vi "ARCO Read Client.vi"() -> ()   [LabVIEW 2017]
uses:
  <vilib>/OPCUA/controls/NodeIds.ctl
  <vilib>/OPCUA/controls/NodeId.ctl
  <vilib>/OPCUA/NI OPC UA Client.lvlib
panel:
  in  "stop":bool
  out "error out":errorcluster
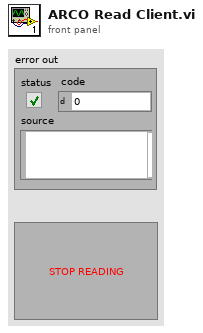
[diagram p1: front panel]
types:
  T1 = cluster{"message mode":enum16{"None", "Sign", "Sign and Encrypt"}, "security":enum16{"Basic256", "Basic128Rsa15"}}
  T2 = typedef "NodeIds.ctl" = T3[]
  T3 = typedef "NodeId.ctl" = string
  T4 = typedef "OPC UA Client Refnum.ctl" = refnum<k21>
  T5 = typedef "Subscription ID.ctl" = u32
  T6 = typedef "Subscription Data Change.ctl" = cluster{"node ID":T3, " value":variant, "timestamp":timestamp, "data type":T7, "status code":T8}
  T7 = typedef "Data Type.ctl" = u16
  T8 = typedef "OPC UA StatusCode.ctl" = u32
  T9 = cluster{"[0]":sgl, "[1]":sgl, "[2]":sgl, "[3]":sgl, "[4]":sgl, "[5]":sgl, "[6]":sgl, "[7]":sgl, "[8]":sgl, "[9]":sgl, "[10]":sgl, "[11]":sgl, "[12]":sgl, "[13]":sgl, "[14]":sgl, "[15]":sgl, "[16]":sgl, "[17]":sgl, "[18]":sgl, "[19]":sgl, "[20]":sgl, "[21]":sgl, "[22]":sgl, "[23]":sgl, "[24]":sgl, "[25]":sgl, "[26]":sgl, "[27]":sgl, "[28]":sgl, "[29]":sgl, "[30]":sgl, "[31]":sgl, "[32]":sgl, "[33]":sgl, "[34]":sgl, "[35]":sgl, "[36]":sgl, "[37]":sgl, "[38]":sgl, "[39]":sgl, "[40]":sgl, "[41]":sgl, "[42]":sgl, "[43]":sgl, "[44]":sgl, "[45]":sgl, "[46]":sgl, "[47]":sgl, "[48]":sgl, "[49]":sgl, "[50]":sgl, "[51]":sgl, "[52]":sgl, "[53]":sgl, "[54]":sgl, "[55]":sgl, "[56]":sgl}
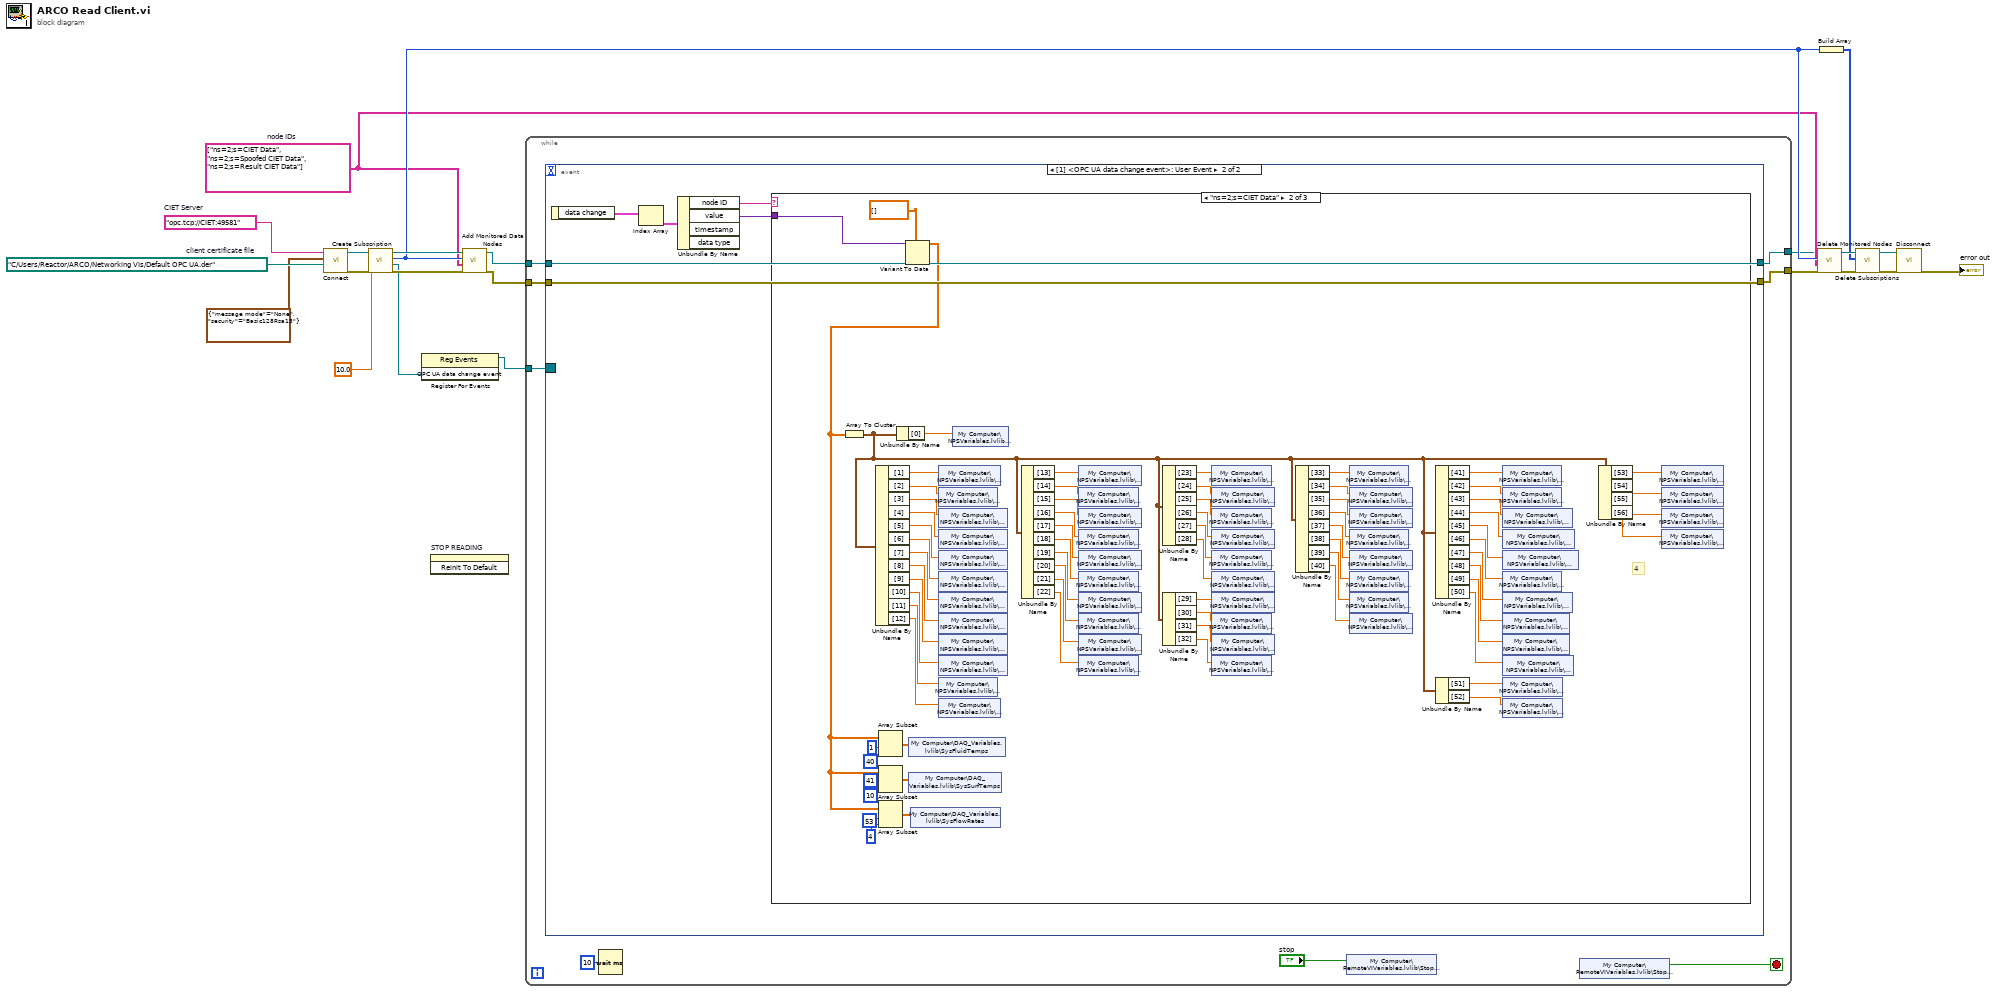
[diagram p0: block diagram]
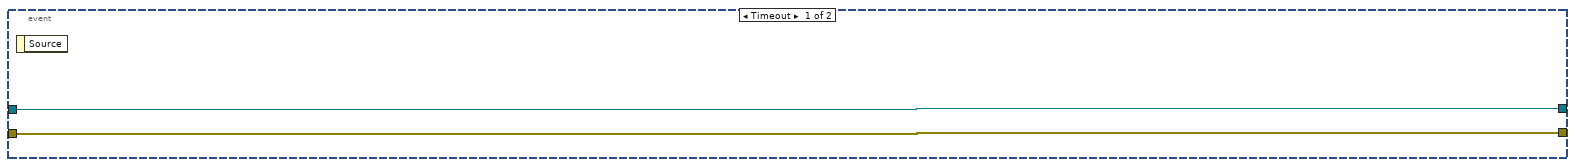
[diagram p2: hidden frame]
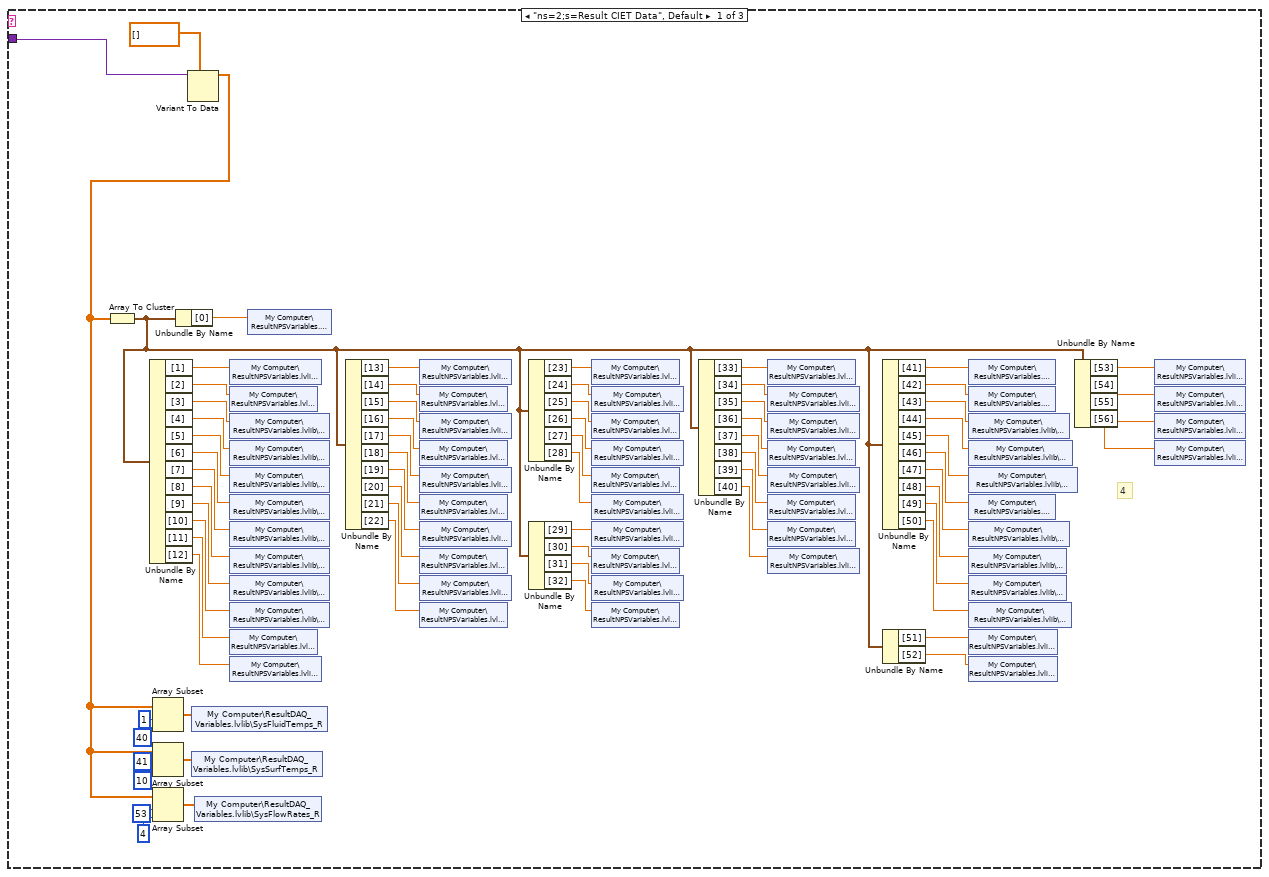
[diagram p3: hidden frame]
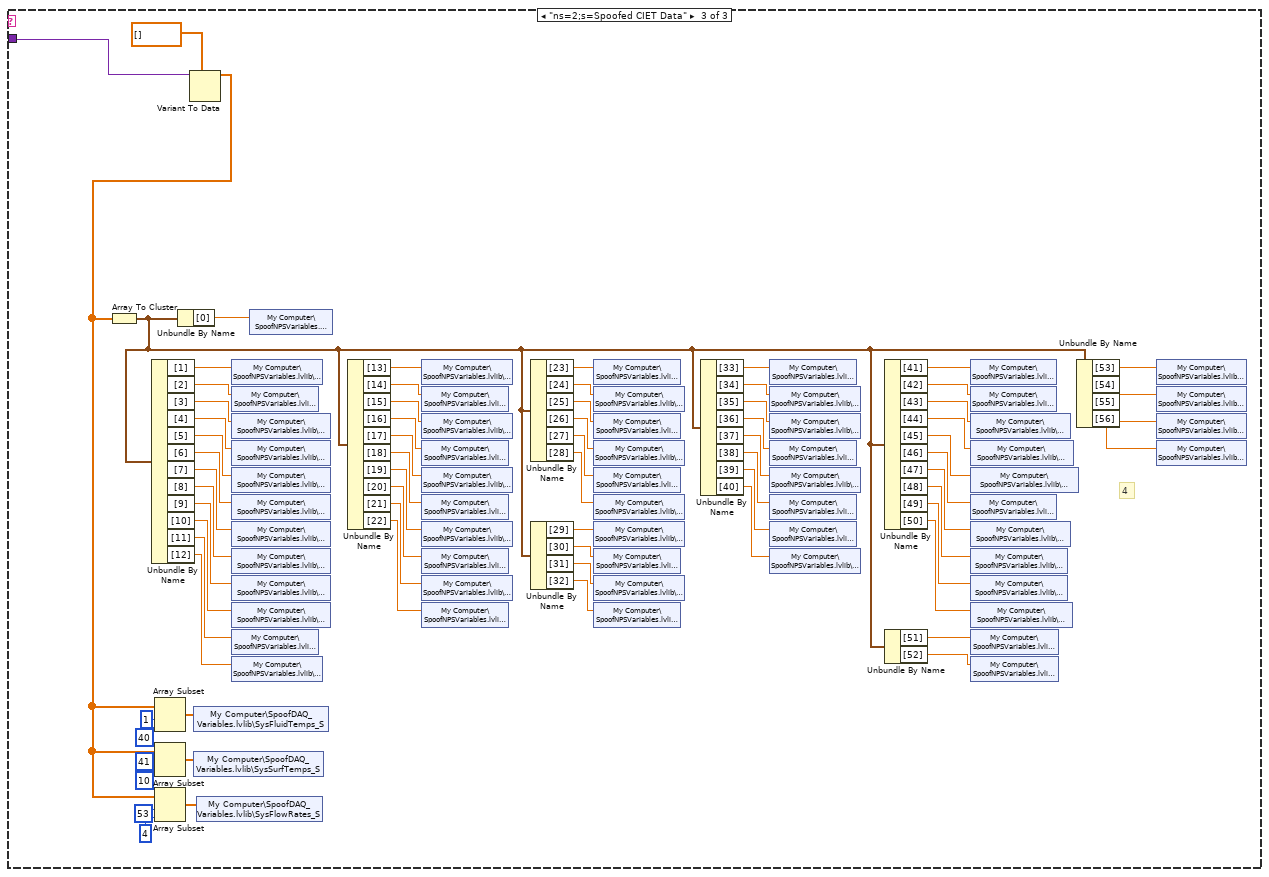
[diagram p4: hidden frame]
diagram:
  w4 = T2 ["ns=2;s=CIET Data", "ns=2;s=Spoofed CIET Data", "ns=2;s=Result CIET Data"]  # node IDs
  w20 = path "C:/Users/Reactor/ARCO/Networking VIs/Default OPC UA.der"  # client certificate file
  w21 = "opc.tcp://CIET:49581"  # CIET Server
  n1 = call <vilib>:"Connect.vi"("client certificate file"=w20, "security policy"=T1 {"message mode"=enum."None", "security"=enum."Basic128Rsa15"}, "server endpoint URL"=w21) -> ("error out"=w16:errorcluster, "OPC UA client refnum out"=w18:T4)  [unwired: 6 in, 1 out]
  n2 = call <vilib>:"Create Subscription.vi"("error in (no error)"=w16, "publishing interval (1000 ms)"=10.0, "OPC UA client refnum in"=w18) -> ("error out"=w15:errorcluster, "OPC UA data change event"=w14:refnum<user-event>, "subscription ID out"=w9:T5, "OPC UA client refnum out"=w17:T4)  [unwired: 4 in, 1 out]
  n3 = register-events(w14) -> (reference out=w7:refnum<event-registration>)  [unwired: 2 in, 1 out]
  n4 = invoke on="STOP READING" class="Bool" method="Reinit To Default"() -> ()  [unwired: 3 in, 3 out]
  n5 = call <vilib>:"Add Monitored Data Nodes.vi"("error in (no error)"=w15, "node IDs"=w4, "subscription ID in"=w9, "OPC UA client refnum in"=w17) -> ("error out"=w5:errorcluster, "OPC UA client refnum out"=w6:T4)  [unwired: 4 in, 2 out]
  n6 = while {
    tunnel: w7 -> [w30]
    tunnel: w6 -> [w29]
    tunnel: w5 -> [w28]
    tunnel: [w27] -> w3
    tunnel: [w26] -> w2
    stop <- w25 stop-if-true
    n7 = event shown="[1] <OPC UA data change event>: User Event" {
      selector: w30 -> [_ _]
      dyn-events: _ -> [_ _]
      timeout: _ -> [_ _]
      tunnel: w29 -> [w32 w36]
      tunnel: [w32 w36] -> w27
      tunnel: w28 -> [w31 w35]
      tunnel: [w31 w35] -> w26
      event Timeout {
        n8 = event-data() -> ()  [unwired: 1 in, 1 out]
      }
      event User Event {
        n9 = event-data() -> ("data change"=w34:T6[])  [unwired: 1 in]
        n10 = Index Array(array=w34) -> (element=w38:T6)  [unwired: 1 in]
        n11 = Unbundle By Name(w38) -> ("node ID"=w33:T3, "value"=w37:variant)  [unwired: 2 out]
        n12 = case shown="\"ns=2;s=CIET Data\"" w33 {
          tunnel: w37 -> [w41 w119 w179]
          frame "ns=2;s=Result CIET Data", Default {
            # "4"
            n13 = Variant To Data(type=sgl[] [], Variant=w41) -> (data=w40:sgl[])  [unwired: 1 in, 1 out]
            n14 = Array To Cluster(array=w40) -> (cluster=w48:T9)
            n15 = Unbundle By Name(w48) -> ("[1]"=w49:sgl, "[2]"=w51:sgl, "[3]"=w52:sgl, "[4]"=w53:sgl, "[5]"=w54:sgl, "[6]"=w55:sgl, "[7]"=w56:sgl, "[8]"=w57:sgl, "[9]"=w58:sgl, "[10]"=w59:sgl, "[11]"=w60:sgl, "[12]"=w61:sgl)
            n16 = Array Subset(array=w40, index=1, length=40) -> (w106:sgl[])
            n17 = Array Subset(array=w40, index=41, length=10) -> (w107:sgl[])
            n18 = Array Subset(array=w40, index=53, length=4) -> (w108:sgl[])
            n19 = Unbundle By Name(w48) -> ("[0]"=w50:sgl)
            n20 = shared-variable "My Computer\\ResultDAQ_Variables.lvlib\\SysFluidTemps_R"(w106) -> ()  [unwired: 1 in, 1 out]
            n21 = shared-variable "My Computer\\ResultDAQ_Variables.lvlib\\SysSurfTemps_R"(w107) -> ()  [unwired: 1 in, 1 out]
            n22 = shared-variable "My Computer\\ResultDAQ_Variables.lvlib\\SysFlowRates_R"(w108) -> ()  [unwired: 1 in, 1 out]
            n23 = shared-variable "My Computer\\ResultNPSVariables.lvlib\\WT-10_R"(w49) -> ()  [unwired: 1 in, 1 out]
            n24 = shared-variable "My Computer\\ResultNPSVariables.lvlib\\BT-11_R"(w51) -> ()  [unwired: 1 in, 1 out]
            n25 = shared-variable "My Computer\\ResultNPSVariables.lvlib\\CX-10-1_R"(w52) -> ()  [unwired: 1 in, 1 out]
            n26 = shared-variable "My Computer\\ResultNPSVariables.lvlib\\CX-10-2_R"(w53) -> ()  [unwired: 1 in, 1 out]
            n27 = shared-variable "My Computer\\ResultNPSVariables.lvlib\\CX-10-3_R"(w54) -> ()  [unwired: 1 in, 1 out]
            n28 = shared-variable "My Computer\\ResultNPSVariables.lvlib\\CX-10-4_R"(w55) -> ()  [unwired: 1 in, 1 out]
            n29 = shared-variable "My Computer\\ResultNPSVariables.lvlib\\CX-11-1_R"(w56) -> ()  [unwired: 1 in, 1 out]
            n30 = shared-variable "My Computer\\ResultNPSVariables.lvlib\\CX-11-2_R"(w57) -> ()  [unwired: 1 in, 1 out]
            n31 = shared-variable "My Computer\\ResultNPSVariables.lvlib\\CX-11-3_R"(w58) -> ()  [unwired: 1 in, 1 out]
            n32 = shared-variable "My Computer\\ResultNPSVariables.lvlib\\CX-11-4_R"(w59) -> ()  [unwired: 1 in, 1 out]
            n33 = shared-variable "My Computer\\ResultNPSVariables.lvlib\\BT-12_R"(w60) -> ()  [unwired: 1 in, 1 out]
            n34 = shared-variable "My Computer\\ResultNPSVariables.lvlib\\WT-13_R"(w61) -> ()  [unwired: 1 in, 1 out]
            n35 = shared-variable "My Computer\\ResultNPSVariables.lvlib\\Time_R"(w50) -> ()  [unwired: 1 in, 1 out]
            n36 = Unbundle By Name(w48) -> ("[13]"=w62:sgl, "[14]"=w63:sgl, "[15]"=w64:sgl, "[16]"=w65:sgl, "[17]"=w66:sgl, "[18]"=w67:sgl, "[19]"=w68:sgl, "[20]"=w69:sgl, "[21]"=w70:sgl, "[22]"=w71:sgl)
            n37 = shared-variable "My Computer\\ResultNPSVariables.lvlib\\WT-20_R"(w62) -> ()  [unwired: 1 in, 1 out]
            n38 = shared-variable "My Computer\\ResultNPSVariables.lvlib\\BT-21_R"(w63) -> ()  [unwired: 1 in, 1 out]
            n39 = shared-variable "My Computer\\ResultNPSVariables.lvlib\\WT-22_R"(w64) -> ()  [unwired: 1 in, 1 out]
            n40 = shared-variable "My Computer\\ResultNPSVariables.lvlib\\BT-23_R"(w65) -> ()  [unwired: 1 in, 1 out]
            n41 = shared-variable "My Computer\\ResultNPSVariables.lvlib\\WT-24_R"(w66) -> ()  [unwired: 1 in, 1 out]
            n42 = shared-variable "My Computer\\ResultNPSVariables.lvlib\\BT-25_R"(w67) -> ()  [unwired: 1 in, 1 out]
            n43 = shared-variable "My Computer\\ResultNPSVariables.lvlib\\WT-26_R"(w68) -> ()  [unwired: 1 in, 1 out]
            n44 = shared-variable "My Computer\\ResultNPSVariables.lvlib\\BT-27_R"(w69) -> ()  [unwired: 1 in, 1 out]
            n45 = shared-variable "My Computer\\ResultNPSVariables.lvlib\\WT-28_R"(w70) -> ()  [unwired: 1 in, 1 out]
            n46 = shared-variable "My Computer\\ResultNPSVariables.lvlib\\BT-29_R"(w71) -> ()  [unwired: 1 in, 1 out]
            n47 = Unbundle By Name(w48) -> ("[23]"=w72:sgl, "[24]"=w73:sgl, "[25]"=w74:sgl, "[26]"=w75:sgl, "[27]"=w76:sgl, "[28]"=w77:sgl)
            n48 = Unbundle By Name(w48) -> ("[29]"=w78:sgl, "[30]"=w79:sgl, "[31]"=w80:sgl, "[32]"=w81:sgl)
            n49 = shared-variable "My Computer\\ResultNPSVariables.lvlib\\BT-30_R"(w72) -> ()  [unwired: 1 in, 1 out]
            n50 = shared-variable "My Computer\\ResultNPSVariables.lvlib\\WT-31_R"(w73) -> ()  [unwired: 1 in, 1 out]
            n51 = shared-variable "My Computer\\ResultNPSVariables.lvlib\\BT-32_R"(w74) -> ()  [unwired: 1 in, 1 out]
            n52 = shared-variable "My Computer\\ResultNPSVariables.lvlib\\WT-33_R"(w75) -> ()  [unwired: 1 in, 1 out]
            n53 = shared-variable "My Computer\\ResultNPSVariables.lvlib\\BT-34_R"(w76) -> ()  [unwired: 1 in, 1 out]
            n54 = shared-variable "My Computer\\ResultNPSVariables.lvlib\\WT-35_R"(w77) -> ()  [unwired: 1 in, 1 out]
            n55 = shared-variable "My Computer\\ResultNPSVariables.lvlib\\WT-40_R"(w78) -> ()  [unwired: 1 in, 1 out]
            n56 = shared-variable "My Computer\\ResultNPSVariables.lvlib\\BT-41_R"(w79) -> ()  [unwired: 1 in, 1 out]
            n57 = shared-variable "My Computer\\ResultNPSVariables.lvlib\\WT-42_R"(w80) -> ()  [unwired: 1 in, 1 out]
            n58 = shared-variable "My Computer\\ResultNPSVariables.lvlib\\BT-43_R"(w81) -> ()  [unwired: 1 in, 1 out]
            n59 = Unbundle By Name(w48) -> ("[33]"=w82:sgl, "[34]"=w83:sgl, "[35]"=w84:sgl, "[36]"=w85:sgl, "[37]"=w86:sgl, "[38]"=w87:sgl, "[39]"=w88:sgl, "[40]"=w89:sgl)
            n60 = shared-variable "My Computer\\ResultNPSVariables.lvlib\\BT-60_R"(w82) -> ()  [unwired: 1 in, 1 out]
            n61 = shared-variable "My Computer\\ResultNPSVariables.lvlib\\WT-61_R"(w83) -> ()  [unwired: 1 in, 1 out]
            n62 = shared-variable "My Computer\\ResultNPSVariables.lvlib\\WT-62_R"(w84) -> ()  [unwired: 1 in, 1 out]
            n63 = shared-variable "My Computer\\ResultNPSVariables.lvlib\\BT-63_R"(w85) -> ()  [unwired: 1 in, 1 out]
            n64 = shared-variable "My Computer\\ResultNPSVariables.lvlib\\WT-64_R"(w86) -> ()  [unwired: 1 in, 1 out]
            n65 = shared-variable "My Computer\\ResultNPSVariables.lvlib\\BT-65_R"(w87) -> ()  [unwired: 1 in, 1 out]
            n66 = shared-variable "My Computer\\ResultNPSVariables.lvlib\\BT-66_R"(w88) -> ()  [unwired: 1 in, 1 out]
            n67 = shared-variable "My Computer\\ResultNPSVariables.lvlib\\WT-67_R"(w89) -> ()  [unwired: 1 in, 1 out]
            n68 = Unbundle By Name(w48) -> ("[41]"=w90:sgl, "[42]"=w91:sgl, "[43]"=w92:sgl, "[44]"=w93:sgl, "[45]"=w94:sgl, "[46]"=w95:sgl, "[47]"=w96:sgl, "[48]"=w97:sgl, "[49]"=w98:sgl, "[50]"=w99:sgl)
            n69 = Unbundle By Name(w48) -> ("[51]"=w100:sgl, "[52]"=w101:sgl)
            n70 = shared-variable "My Computer\\ResultNPSVariables.lvlib\\ST-10_R"(w90) -> ()  [unwired: 1 in, 1 out]
            n71 = shared-variable "My Computer\\ResultNPSVariables.lvlib\\ST-11_R"(w91) -> ()  [unwired: 1 in, 1 out]
            n72 = shared-variable "My Computer\\ResultNPSVariables.lvlib\\ST-12-N_R"(w92) -> ()  [unwired: 1 in, 1 out]
            n73 = shared-variable "My Computer\\ResultNPSVariables.lvlib\\ST-12-SE_R"(w93) -> ()  [unwired: 1 in, 1 out]
            n74 = shared-variable "My Computer\\ResultNPSVariables.lvlib\\ST-12-SW_R"(w94) -> ()  [unwired: 1 in, 1 out]
            n75 = shared-variable "My Computer\\ResultNPSVariables.lvlib\\ST-13_R"(w95) -> ()  [unwired: 1 in, 1 out]
            n76 = shared-variable "My Computer\\ResultNPSVariables.lvlib\\ST-14-N_R"(w96) -> ()  [unwired: 1 in, 1 out]
            n77 = shared-variable "My Computer\\ResultNPSVariables.lvlib\\ST-14-E_R"(w97) -> ()  [unwired: 1 in, 1 out]
            n78 = shared-variable "My Computer\\ResultNPSVariables.lvlib\\ST-14-S_R"(w98) -> ()  [unwired: 1 in, 1 out]
            n79 = shared-variable "My Computer\\ResultNPSVariables.lvlib\\ST-14-W_R"(w99) -> ()  [unwired: 1 in, 1 out]
            n80 = shared-variable "My Computer\\ResultNPSVariables.lvlib\\AT-01_R"(w100) -> ()  [unwired: 1 in, 1 out]
            n81 = shared-variable "My Computer\\ResultNPSVariables.lvlib\\AT-02_R"(w101) -> ()  [unwired: 1 in, 1 out]
            n82 = Unbundle By Name(w48) -> ("[53]"=w102:sgl, "[54]"=w103:sgl, "[55]"=w104:sgl, "[56]"=w105:sgl)
            n83 = shared-variable "My Computer\\ResultNPSVariables.lvlib\\FM-20_R"(w102) -> ()  [unwired: 1 in, 1 out]
            n84 = shared-variable "My Computer\\ResultNPSVariables.lvlib\\FM-30_R"(w103) -> ()  [unwired: 1 in, 1 out]
            n85 = shared-variable "My Computer\\ResultNPSVariables.lvlib\\FM-40_R"(w104) -> ()  [unwired: 1 in, 1 out]
            n86 = shared-variable "My Computer\\ResultNPSVariables.lvlib\\FM-60_R"(w105) -> ()  [unwired: 1 in, 1 out]
          }
          frame "ns=2;s=CIET Data" {
            # "4"
            n87 = Variant To Data(type=sgl[] [], Variant=w119) -> (data=w116:sgl[])  [unwired: 1 in, 1 out]
            n88 = Array To Cluster(array=w116) -> (cluster=w115:T9)
            n89 = Unbundle By Name(w115) -> ("[1]"=w118:sgl, "[2]"=w121:sgl, "[3]"=w122:sgl, "[4]"=w123:sgl, "[5]"=w124:sgl, "[6]"=w125:sgl, "[7]"=w126:sgl, "[8]"=w127:sgl, "[9]"=w128:sgl, "[10]"=w129:sgl, "[11]"=w130:sgl, "[12]"=w131:sgl)
            n90 = Array Subset(array=w116, index=1, length=40) -> (w176:sgl[])
            n91 = Array Subset(array=w116, index=41, length=10) -> (w177:sgl[])
            n92 = Array Subset(array=w116, index=53, length=4) -> (w178:sgl[])
            n93 = Unbundle By Name(w115) -> ("[0]"=w120:sgl)
            n94 = shared-variable "My Computer\\DAQ_Variables.lvlib\\SysFluidTemps"(w176) -> ()  [unwired: 1 in, 1 out]
            n95 = shared-variable "My Computer\\DAQ_Variables.lvlib\\SysSurfTemps"(w177) -> ()  [unwired: 1 in, 1 out]
            n96 = shared-variable "My Computer\\DAQ_Variables.lvlib\\SysFlowRates"(w178) -> ()  [unwired: 1 in, 1 out]
            n97 = shared-variable "My Computer\\NPSVariables.lvlib\\WT-10"(w118) -> ()  [unwired: 1 in, 1 out]
            n98 = shared-variable "My Computer\\NPSVariables.lvlib\\BT-11"(w121) -> ()  [unwired: 1 in, 1 out]
            n99 = shared-variable "My Computer\\NPSVariables.lvlib\\CX-10-1"(w122) -> ()  [unwired: 1 in, 1 out]
            n100 = shared-variable "My Computer\\NPSVariables.lvlib\\CX-10-2"(w123) -> ()  [unwired: 1 in, 1 out]
            n101 = shared-variable "My Computer\\NPSVariables.lvlib\\CX-10-3"(w124) -> ()  [unwired: 1 in, 1 out]
            n102 = shared-variable "My Computer\\NPSVariables.lvlib\\CX-10-4"(w125) -> ()  [unwired: 1 in, 1 out]
            n103 = shared-variable "My Computer\\NPSVariables.lvlib\\CX-11-1"(w126) -> ()  [unwired: 1 in, 1 out]
            n104 = shared-variable "My Computer\\NPSVariables.lvlib\\CX-11-2"(w127) -> ()  [unwired: 1 in, 1 out]
            n105 = shared-variable "My Computer\\NPSVariables.lvlib\\CX-11-3"(w128) -> ()  [unwired: 1 in, 1 out]
            n106 = shared-variable "My Computer\\NPSVariables.lvlib\\CX-11-4"(w129) -> ()  [unwired: 1 in, 1 out]
            n107 = shared-variable "My Computer\\NPSVariables.lvlib\\BT-12"(w130) -> ()  [unwired: 1 in, 1 out]
            n108 = shared-variable "My Computer\\NPSVariables.lvlib\\WT-13"(w131) -> ()  [unwired: 1 in, 1 out]
            n109 = shared-variable "My Computer\\NPSVariables.lvlib\\Time"(w120) -> ()  [unwired: 1 in, 1 out]
            n110 = Unbundle By Name(w115) -> ("[13]"=w132:sgl, "[14]"=w133:sgl, "[15]"=w134:sgl, "[16]"=w135:sgl, "[17]"=w136:sgl, "[18]"=w137:sgl, "[19]"=w138:sgl, "[20]"=w139:sgl, "[21]"=w140:sgl, "[22]"=w141:sgl)
            n111 = shared-variable "My Computer\\NPSVariables.lvlib\\WT-20"(w132) -> ()  [unwired: 1 in, 1 out]
            n112 = shared-variable "My Computer\\NPSVariables.lvlib\\BT-21"(w133) -> ()  [unwired: 1 in, 1 out]
            n113 = shared-variable "My Computer\\NPSVariables.lvlib\\WT-22"(w134) -> ()  [unwired: 1 in, 1 out]
            n114 = shared-variable "My Computer\\NPSVariables.lvlib\\BT-23"(w135) -> ()  [unwired: 1 in, 1 out]
            n115 = shared-variable "My Computer\\NPSVariables.lvlib\\WT-24"(w136) -> ()  [unwired: 1 in, 1 out]
            n116 = shared-variable "My Computer\\NPSVariables.lvlib\\BT-25"(w137) -> ()  [unwired: 1 in, 1 out]
            n117 = shared-variable "My Computer\\NPSVariables.lvlib\\WT-26"(w138) -> ()  [unwired: 1 in, 1 out]
            n118 = shared-variable "My Computer\\NPSVariables.lvlib\\BT-27"(w139) -> ()  [unwired: 1 in, 1 out]
            n119 = shared-variable "My Computer\\NPSVariables.lvlib\\WT-28"(w140) -> ()  [unwired: 1 in, 1 out]
            n120 = shared-variable "My Computer\\NPSVariables.lvlib\\BT-29"(w141) -> ()  [unwired: 1 in, 1 out]
            n121 = Unbundle By Name(w115) -> ("[23]"=w142:sgl, "[24]"=w143:sgl, "[25]"=w144:sgl, "[26]"=w145:sgl, "[27]"=w146:sgl, "[28]"=w147:sgl)
            n122 = Unbundle By Name(w115) -> ("[29]"=w148:sgl, "[30]"=w149:sgl, "[31]"=w150:sgl, "[32]"=w151:sgl)
            n123 = shared-variable "My Computer\\NPSVariables.lvlib\\BT-30"(w142) -> ()  [unwired: 1 in, 1 out]
            n124 = shared-variable "My Computer\\NPSVariables.lvlib\\WT-31"(w143) -> ()  [unwired: 1 in, 1 out]
            n125 = shared-variable "My Computer\\NPSVariables.lvlib\\BT-32"(w144) -> ()  [unwired: 1 in, 1 out]
            n126 = shared-variable "My Computer\\NPSVariables.lvlib\\WT-33"(w145) -> ()  [unwired: 1 in, 1 out]
            n127 = shared-variable "My Computer\\NPSVariables.lvlib\\BT-34"(w146) -> ()  [unwired: 1 in, 1 out]
            n128 = shared-variable "My Computer\\NPSVariables.lvlib\\WT-35"(w147) -> ()  [unwired: 1 in, 1 out]
            n129 = shared-variable "My Computer\\NPSVariables.lvlib\\WT-40"(w148) -> ()  [unwired: 1 in, 1 out]
            n130 = shared-variable "My Computer\\NPSVariables.lvlib\\BT-41"(w149) -> ()  [unwired: 1 in, 1 out]
            n131 = shared-variable "My Computer\\NPSVariables.lvlib\\WT-42"(w150) -> ()  [unwired: 1 in, 1 out]
            n132 = shared-variable "My Computer\\NPSVariables.lvlib\\BT-43"(w151) -> ()  [unwired: 1 in, 1 out]
            n133 = Unbundle By Name(w115) -> ("[33]"=w152:sgl, "[34]"=w153:sgl, "[35]"=w154:sgl, "[36]"=w155:sgl, "[37]"=w156:sgl, "[38]"=w157:sgl, "[39]"=w158:sgl, "[40]"=w159:sgl)
            n134 = shared-variable "My Computer\\NPSVariables.lvlib\\BT-60"(w152) -> ()  [unwired: 1 in, 1 out]
            n135 = shared-variable "My Computer\\NPSVariables.lvlib\\WT-61"(w153) -> ()  [unwired: 1 in, 1 out]
            n136 = shared-variable "My Computer\\NPSVariables.lvlib\\WT-62"(w154) -> ()  [unwired: 1 in, 1 out]
            n137 = shared-variable "My Computer\\NPSVariables.lvlib\\BT-63"(w155) -> ()  [unwired: 1 in, 1 out]
            n138 = shared-variable "My Computer\\NPSVariables.lvlib\\WT-64"(w156) -> ()  [unwired: 1 in, 1 out]
            n139 = shared-variable "My Computer\\NPSVariables.lvlib\\BT-65"(w157) -> ()  [unwired: 1 in, 1 out]
            n140 = shared-variable "My Computer\\NPSVariables.lvlib\\BT-66"(w158) -> ()  [unwired: 1 in, 1 out]
            n141 = shared-variable "My Computer\\NPSVariables.lvlib\\WT-67"(w159) -> ()  [unwired: 1 in, 1 out]
            n142 = Unbundle By Name(w115) -> ("[41]"=w160:sgl, "[42]"=w161:sgl, "[43]"=w162:sgl, "[44]"=w163:sgl, "[45]"=w164:sgl, "[46]"=w165:sgl, "[47]"=w166:sgl, "[48]"=w167:sgl, "[49]"=w168:sgl, "[50]"=w169:sgl)
            n143 = Unbundle By Name(w115) -> ("[51]"=w170:sgl, "[52]"=w171:sgl)
            n144 = shared-variable "My Computer\\NPSVariables.lvlib\\ST-10"(w160) -> ()  [unwired: 1 in, 1 out]
            n145 = shared-variable "My Computer\\NPSVariables.lvlib\\ST-11"(w161) -> ()  [unwired: 1 in, 1 out]
            n146 = shared-variable "My Computer\\NPSVariables.lvlib\\ST-12-N"(w162) -> ()  [unwired: 1 in, 1 out]
            n147 = shared-variable "My Computer\\NPSVariables.lvlib\\ST-12-SE"(w163) -> ()  [unwired: 1 in, 1 out]
            n148 = shared-variable "My Computer\\NPSVariables.lvlib\\ST-12-SW"(w164) -> ()  [unwired: 1 in, 1 out]
            n149 = shared-variable "My Computer\\NPSVariables.lvlib\\ST-13"(w165) -> ()  [unwired: 1 in, 1 out]
            n150 = shared-variable "My Computer\\NPSVariables.lvlib\\ST-14-N"(w166) -> ()  [unwired: 1 in, 1 out]
            n151 = shared-variable "My Computer\\NPSVariables.lvlib\\ST-14-E"(w167) -> ()  [unwired: 1 in, 1 out]
            n152 = shared-variable "My Computer\\NPSVariables.lvlib\\ST-14-S"(w168) -> ()  [unwired: 1 in, 1 out]
            n153 = shared-variable "My Computer\\NPSVariables.lvlib\\ST-14-W"(w169) -> ()  [unwired: 1 in, 1 out]
            n154 = shared-variable "My Computer\\NPSVariables.lvlib\\AT-01"(w170) -> ()  [unwired: 1 in, 1 out]
            n155 = shared-variable "My Computer\\NPSVariables.lvlib\\AT-02"(w171) -> ()  [unwired: 1 in, 1 out]
            n156 = Unbundle By Name(w115) -> ("[53]"=w172:sgl, "[54]"=w173:sgl, "[55]"=w174:sgl, "[56]"=w175:sgl)
            n157 = shared-variable "My Computer\\NPSVariables.lvlib\\FM-20"(w172) -> ()  [unwired: 1 in, 1 out]
            n158 = shared-variable "My Computer\\NPSVariables.lvlib\\FM-30"(w173) -> ()  [unwired: 1 in, 1 out]
            n159 = shared-variable "My Computer\\NPSVariables.lvlib\\FM-40"(w174) -> ()  [unwired: 1 in, 1 out]
            n160 = shared-variable "My Computer\\NPSVariables.lvlib\\FM-60"(w175) -> ()  [unwired: 1 in, 1 out]
          }
          frame "ns=2;s=Spoofed CIET Data" {
            # "4"
            n161 = Variant To Data(type=sgl[] [], Variant=w179) -> (data=w181:sgl[])  [unwired: 1 in, 1 out]
            n162 = Array To Cluster(array=w181) -> (cluster=w188:T9)
            n163 = Unbundle By Name(w188) -> ("[1]"=w189:sgl, "[2]"=w191:sgl, "[3]"=w192:sgl, "[4]"=w193:sgl, "[5]"=w194:sgl, "[6]"=w195:sgl, "[7]"=w196:sgl, "[8]"=w197:sgl, "[9]"=w198:sgl, "[10]"=w199:sgl, "[11]"=w200:sgl, "[12]"=w201:sgl)
            n164 = Array Subset(array=w181, index=1, length=40) -> (w246:sgl[])
            n165 = Array Subset(array=w181, index=41, length=10) -> (w247:sgl[])
            n166 = Array Subset(array=w181, index=53, length=4) -> (w248:sgl[])
            n167 = Unbundle By Name(w188) -> ("[0]"=w190:sgl)
            n168 = shared-variable "My Computer\\SpoofDAQ_Variables.lvlib\\SysFluidTemps_S"(w246) -> ()  [unwired: 1 in, 1 out]
            n169 = shared-variable "My Computer\\SpoofDAQ_Variables.lvlib\\SysSurfTemps_S"(w247) -> ()  [unwired: 1 in, 1 out]
            n170 = shared-variable "My Computer\\SpoofDAQ_Variables.lvlib\\SysFlowRates_S"(w248) -> ()  [unwired: 1 in, 1 out]
            n171 = shared-variable "My Computer\\SpoofNPSVariables.lvlib\\WT-10_S"(w189) -> ()  [unwired: 1 in, 1 out]
            n172 = shared-variable "My Computer\\SpoofNPSVariables.lvlib\\BT-11_S"(w191) -> ()  [unwired: 1 in, 1 out]
            n173 = shared-variable "My Computer\\SpoofNPSVariables.lvlib\\CX-10-1_S"(w192) -> ()  [unwired: 1 in, 1 out]
            n174 = shared-variable "My Computer\\SpoofNPSVariables.lvlib\\CX-10-2_S"(w193) -> ()  [unwired: 1 in, 1 out]
            n175 = shared-variable "My Computer\\SpoofNPSVariables.lvlib\\CX-10-3_S"(w194) -> ()  [unwired: 1 in, 1 out]
            n176 = shared-variable "My Computer\\SpoofNPSVariables.lvlib\\CX-10-4_S"(w195) -> ()  [unwired: 1 in, 1 out]
            n177 = shared-variable "My Computer\\SpoofNPSVariables.lvlib\\CX-11-1_S"(w196) -> ()  [unwired: 1 in, 1 out]
            n178 = shared-variable "My Computer\\SpoofNPSVariables.lvlib\\CX-11-2_S"(w197) -> ()  [unwired: 1 in, 1 out]
            n179 = shared-variable "My Computer\\SpoofNPSVariables.lvlib\\CX-11-3_S"(w198) -> ()  [unwired: 1 in, 1 out]
            n180 = shared-variable "My Computer\\SpoofNPSVariables.lvlib\\CX-11-4_S"(w199) -> ()  [unwired: 1 in, 1 out]
            n181 = shared-variable "My Computer\\SpoofNPSVariables.lvlib\\BT-12_S"(w200) -> ()  [unwired: 1 in, 1 out]
            n182 = shared-variable "My Computer\\SpoofNPSVariables.lvlib\\WT-13_S"(w201) -> ()  [unwired: 1 in, 1 out]
            n183 = shared-variable "My Computer\\SpoofNPSVariables.lvlib\\Time_S"(w190) -> ()  [unwired: 1 in, 1 out]
            n184 = Unbundle By Name(w188) -> ("[13]"=w202:sgl, "[14]"=w203:sgl, "[15]"=w204:sgl, "[16]"=w205:sgl, "[17]"=w206:sgl, "[18]"=w207:sgl, "[19]"=w208:sgl, "[20]"=w209:sgl, "[21]"=w210:sgl, "[22]"=w211:sgl)
            n185 = shared-variable "My Computer\\SpoofNPSVariables.lvlib\\WT-20_S"(w202) -> ()  [unwired: 1 in, 1 out]
            n186 = shared-variable "My Computer\\SpoofNPSVariables.lvlib\\BT-21_S"(w203) -> ()  [unwired: 1 in, 1 out]
            n187 = shared-variable "My Computer\\SpoofNPSVariables.lvlib\\WT-22_S"(w204) -> ()  [unwired: 1 in, 1 out]
            n188 = shared-variable "My Computer\\SpoofNPSVariables.lvlib\\BT-23_S"(w205) -> ()  [unwired: 1 in, 1 out]
            n189 = shared-variable "My Computer\\SpoofNPSVariables.lvlib\\WT-24_S"(w206) -> ()  [unwired: 1 in, 1 out]
            n190 = shared-variable "My Computer\\SpoofNPSVariables.lvlib\\BT-25_S"(w207) -> ()  [unwired: 1 in, 1 out]
            n191 = shared-variable "My Computer\\SpoofNPSVariables.lvlib\\WT-26_S"(w208) -> ()  [unwired: 1 in, 1 out]
            n192 = shared-variable "My Computer\\SpoofNPSVariables.lvlib\\BT-27_S"(w209) -> ()  [unwired: 1 in, 1 out]
            n193 = shared-variable "My Computer\\SpoofNPSVariables.lvlib\\WT-28_S"(w210) -> ()  [unwired: 1 in, 1 out]
            n194 = shared-variable "My Computer\\SpoofNPSVariables.lvlib\\BT-29_S"(w211) -> ()  [unwired: 1 in, 1 out]
            n195 = Unbundle By Name(w188) -> ("[23]"=w212:sgl, "[24]"=w213:sgl, "[25]"=w214:sgl, "[26]"=w215:sgl, "[27]"=w216:sgl, "[28]"=w217:sgl)
            n196 = Unbundle By Name(w188) -> ("[29]"=w218:sgl, "[30]"=w219:sgl, "[31]"=w220:sgl, "[32]"=w221:sgl)
            n197 = shared-variable "My Computer\\SpoofNPSVariables.lvlib\\BT-30_S"(w212) -> ()  [unwired: 1 in, 1 out]
            n198 = shared-variable "My Computer\\SpoofNPSVariables.lvlib\\WT-31_S"(w213) -> ()  [unwired: 1 in, 1 out]
            n199 = shared-variable "My Computer\\SpoofNPSVariables.lvlib\\BT-32_S"(w214) -> ()  [unwired: 1 in, 1 out]
            n200 = shared-variable "My Computer\\SpoofNPSVariables.lvlib\\WT-33_S"(w215) -> ()  [unwired: 1 in, 1 out]
            n201 = shared-variable "My Computer\\SpoofNPSVariables.lvlib\\BT-34_S"(w216) -> ()  [unwired: 1 in, 1 out]
            n202 = shared-variable "My Computer\\SpoofNPSVariables.lvlib\\WT-35_S"(w217) -> ()  [unwired: 1 in, 1 out]
            n203 = shared-variable "My Computer\\SpoofNPSVariables.lvlib\\WT-40_S"(w218) -> ()  [unwired: 1 in, 1 out]
            n204 = shared-variable "My Computer\\SpoofNPSVariables.lvlib\\BT-41_S"(w219) -> ()  [unwired: 1 in, 1 out]
            n205 = shared-variable "My Computer\\SpoofNPSVariables.lvlib\\WT-42_S"(w220) -> ()  [unwired: 1 in, 1 out]
            n206 = shared-variable "My Computer\\SpoofNPSVariables.lvlib\\BT-43_S"(w221) -> ()  [unwired: 1 in, 1 out]
            n207 = Unbundle By Name(w188) -> ("[33]"=w222:sgl, "[34]"=w223:sgl, "[35]"=w224:sgl, "[36]"=w225:sgl, "[37]"=w226:sgl, "[38]"=w227:sgl, "[39]"=w228:sgl, "[40]"=w229:sgl)
            n208 = shared-variable "My Computer\\SpoofNPSVariables.lvlib\\BT-60_S"(w222) -> ()  [unwired: 1 in, 1 out]
            n209 = shared-variable "My Computer\\SpoofNPSVariables.lvlib\\WT-61_S"(w223) -> ()  [unwired: 1 in, 1 out]
            n210 = shared-variable "My Computer\\SpoofNPSVariables.lvlib\\WT-62_S"(w224) -> ()  [unwired: 1 in, 1 out]
            n211 = shared-variable "My Computer\\SpoofNPSVariables.lvlib\\BT-63_S"(w225) -> ()  [unwired: 1 in, 1 out]
            n212 = shared-variable "My Computer\\SpoofNPSVariables.lvlib\\WT-64_S"(w226) -> ()  [unwired: 1 in, 1 out]
            n213 = shared-variable "My Computer\\SpoofNPSVariables.lvlib\\BT-65_S"(w227) -> ()  [unwired: 1 in, 1 out]
            n214 = shared-variable "My Computer\\SpoofNPSVariables.lvlib\\BT-66_S"(w228) -> ()  [unwired: 1 in, 1 out]
            n215 = shared-variable "My Computer\\SpoofNPSVariables.lvlib\\WT-67_S"(w229) -> ()  [unwired: 1 in, 1 out]
            n216 = Unbundle By Name(w188) -> ("[41]"=w230:sgl, "[42]"=w231:sgl, "[43]"=w232:sgl, "[44]"=w233:sgl, "[45]"=w234:sgl, "[46]"=w235:sgl, "[47]"=w236:sgl, "[48]"=w237:sgl, "[49]"=w238:sgl, "[50]"=w239:sgl)
            n217 = Unbundle By Name(w188) -> ("[51]"=w240:sgl, "[52]"=w241:sgl)
            n218 = shared-variable "My Computer\\SpoofNPSVariables.lvlib\\ST-10_S"(w230) -> ()  [unwired: 1 in, 1 out]
            n219 = shared-variable "My Computer\\SpoofNPSVariables.lvlib\\ST-11_S"(w231) -> ()  [unwired: 1 in, 1 out]
            n220 = shared-variable "My Computer\\SpoofNPSVariables.lvlib\\ST-12-N_S"(w232) -> ()  [unwired: 1 in, 1 out]
            n221 = shared-variable "My Computer\\SpoofNPSVariables.lvlib\\ST-12-SE_S"(w233) -> ()  [unwired: 1 in, 1 out]
            n222 = shared-variable "My Computer\\SpoofNPSVariables.lvlib\\ST-12-SW_S"(w234) -> ()  [unwired: 1 in, 1 out]
            n223 = shared-variable "My Computer\\SpoofNPSVariables.lvlib\\ST-13_S"(w235) -> ()  [unwired: 1 in, 1 out]
            n224 = shared-variable "My Computer\\SpoofNPSVariables.lvlib\\ST-14-N_S"(w236) -> ()  [unwired: 1 in, 1 out]
            n225 = shared-variable "My Computer\\SpoofNPSVariables.lvlib\\ST-14-E_S"(w237) -> ()  [unwired: 1 in, 1 out]
            n226 = shared-variable "My Computer\\SpoofNPSVariables.lvlib\\ST-14-S_S"(w238) -> ()  [unwired: 1 in, 1 out]
            n227 = shared-variable "My Computer\\SpoofNPSVariables.lvlib\\ST-14-W_S"(w239) -> ()  [unwired: 1 in, 1 out]
            n228 = shared-variable "My Computer\\SpoofNPSVariables.lvlib\\AT-01_S"(w240) -> ()  [unwired: 1 in, 1 out]
            n229 = shared-variable "My Computer\\SpoofNPSVariables.lvlib\\AT-02_S"(w241) -> ()  [unwired: 1 in, 1 out]
            n230 = Unbundle By Name(w188) -> ("[53]"=w242:sgl, "[54]"=w243:sgl, "[55]"=w244:sgl, "[56]"=w245:sgl)
            n231 = shared-variable "My Computer\\SpoofNPSVariables.lvlib\\FM-20_S"(w242) -> ()  [unwired: 1 in, 1 out]
            n232 = shared-variable "My Computer\\SpoofNPSVariables.lvlib\\FM-30_S"(w243) -> ()  [unwired: 1 in, 1 out]
            n233 = shared-variable "My Computer\\SpoofNPSVariables.lvlib\\FM-40_S"(w244) -> ()  [unwired: 1 in, 1 out]
            n234 = shared-variable "My Computer\\SpoofNPSVariables.lvlib\\FM-60_S"(w245) -> ()  [unwired: 1 in, 1 out]
          }
        }
      }
    }
    n235 = Wait (ms)(milliseconds to wait=u32 10) -> ()  [unwired: 1 out]
    n236 = shared-variable "My Computer\\RemoteVIVariables.lvlib\\Stop Reading"("stop") -> ()  [unwired: 1 in, 1 out]
    n237 = shared-variable "My Computer\\RemoteVIVariables.lvlib\\Stop Reading"() -> (w25:bool)  [unwired: 1 in, 1 out]
  }
  n238 = call <vilib>:"Delete Monitored Nodes.vi"("error in (no error)"=w2, "node IDs"=w4, "subscription ID in"=w9, "OPC UA client refnum in"=w3) -> ("error out"=w10:errorcluster, "OPC UA client refnum out"=w11:T4)  [unwired: 3 in, 3 out]
  n239 = Build Array(w9) -> (w8:T5[])
  n240 = call <vilib>:"Delete Subscriptions.vi"("error in (no error)"=w10, "subscription IDs"=w8, "OPC UA client refnum in"=w11) -> ("error out"=w12:errorcluster, "OPC UA client refnum out"=w13:T4)  [unwired: 6 in, 1 out]
  n241 = call <vilib>:"Disconnect.vi"("error in (no error)"=w12, "OPC UA client refnum in"=w13) -> ("error out"=→"error out":errorcluster)  [unwired: 9 in]
